vi "Open file in ImageJ.vi"(8 "Process Index":i32, 9 "Na/Rb (0/1)":u8, 11 "Current File Num":i32) -> ()   [LabVIEW 2015]
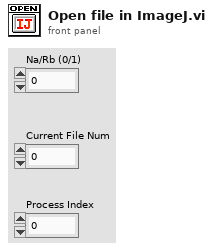
[diagram p1: front panel]
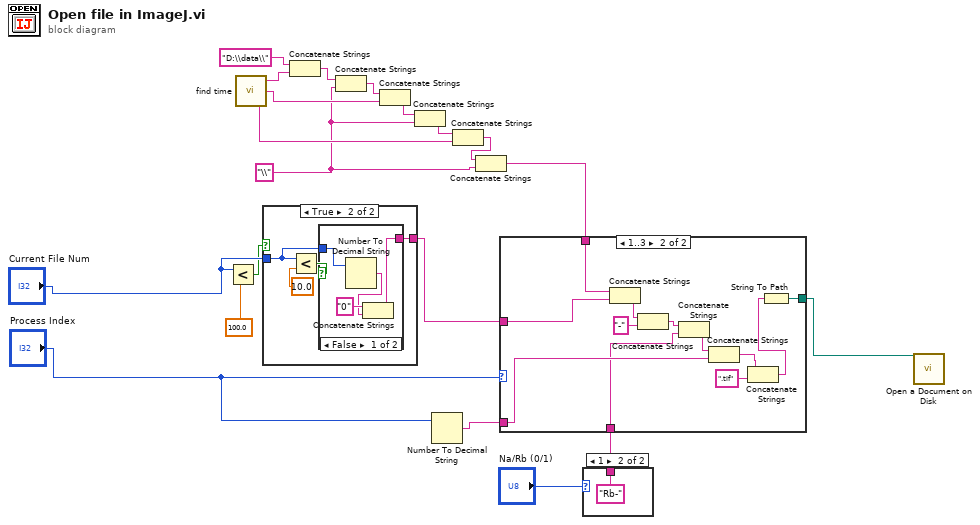
[diagram p0: block diagram]
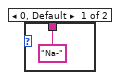
[diagram p2: hidden frame]
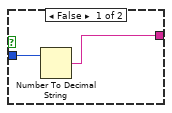
[diagram p3: hidden frame]
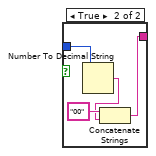
[diagram p4: hidden frame]
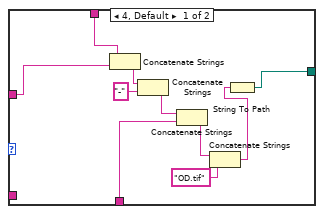
[diagram p5: hidden frame]
diagram:
  w9 = "\\" ("字符串")
  n1 = Less?(x="Current File Num", y=100.0) -> (x < y?=w6:bool)
  n2 = call "find time.vi"() -> ("day"=w11:string, "month"=w14:string, "year"=w17:string)  [unwired: 3 in]
  n3 = case shown="True" w6 {
    tunnel: "Current File Num" -> [w22 w24]
    tunnel: [w21 w23] -> w5
    frame False {
      n4 = Number To Decimal String(number=w22) -> (decimal integer string=w21:string)  [unwired: 1 in]
    }
    frame True {
      n5 = Less?(x=w24, y=10.0) -> (x < y?=w25:bool)
      n6 = case shown="False" w25 {
        tunnel: w24 -> [w29 w34]
        tunnel: [w27 w31] -> w23
        frame False {
          n7 = Number To Decimal String(number=w29) -> (decimal integer string=w28:string)  [unwired: 1 in]
          n8 = Concatenate Strings("0" ("字符串"), w28) -> (w27:string)
        }
        frame True {
          n9 = Number To Decimal String(number=w34) -> (decimal integer string=w32:string)  [unwired: 1 in]
          n10 = Concatenate Strings("00" ("字符串"), w32) -> (w31:string)
        }
      }
    }
  }
  n11 = Concatenate Strings("D:\\data\\", w17) -> (w16:string)
  n12 = Concatenate Strings(w16, w9) -> (w15:string)
  n13 = Concatenate Strings(w15, w14) -> (w13:string)
  n14 = Concatenate Strings(w13, w9) -> (w12:string)
  n15 = Number To Decimal String(number="Process Index") -> (decimal integer string=w8:string)  [unwired: 1 in]
  n16 = Concatenate Strings(w12, w11) -> (w10:string)
  n17 = Concatenate Strings(w10, w9) -> (w4:string)
  n18 = case shown="1" "Na/Rb (0/1)" {
    tunnel: ["Na-" ("string") "Rb-" ("string")] -> w1
    frame 0, Default {
    }
    frame 1 {
    }
  }
  n19 = case shown="1..3" "Process Index" {
    tunnel: [w41 w58] -> w3
    tunnel: w5 -> [w44 w57]
    tunnel: w8 -> [_ w54]
    tunnel: w4 -> [w40 w53]
    tunnel: w1 -> [w38 w48]
    frame 4, Default {
      n20 = Concatenate Strings(w40, w44) -> (w46:string)
      n21 = Concatenate Strings(w46, "-" ("字符串")) -> (w39:string)
      n22 = Concatenate Strings(w39, w38) -> (w37:string)
      n23 = Concatenate Strings(w37, "OD.tif" ("字符串")) -> (w42:string)
      n24 = String To Path(string=w42) -> (path=w41:path)
    }
    frame 1..3 {
      n25 = Concatenate Strings(w53, w57) -> (w56:string)
      n26 = Concatenate Strings(w56, "-" ("字符串")) -> (w49:string)
      n27 = Concatenate Strings(w49, w48) -> (w47:string)
      n28 = Concatenate Strings(w47, w54) -> (w51:string)
      n29 = Concatenate Strings(w51, ".tif" ("字符串")) -> (w50:string)
      n30 = String To Path(string=w50) -> (path=w58:path)
    }
  }
  n31 = call <vilib>:"Open a Document on Disk.vi"("document path"=w3) -> ()  [unwired: 6 in, 1 out]
